vi "AddWatchdog.vi"(8 "error in (no error)":errorcluster, 10 "Watchdog":refnum<data-value>, 11 "Pound in":refnum<class "Pound.lvclass">) -> (0 "error out":errorcluster, 3 "Pound out":refnum<class "Pound.lvclass">)   [LabVIEW 2017, in "Pound.lvclass"]
doc: "Add a watchdog to the pack."
uses:
  <vilib>/NI/Software Watchdog/Pound/Pound.lvclass
  <vilib>/NI/Software Watchdog/Watchdog/Watchdog.lvclass
  <vilib>/NI/Software Watchdog/Pound/Pound.lvclass/Pound.ctl
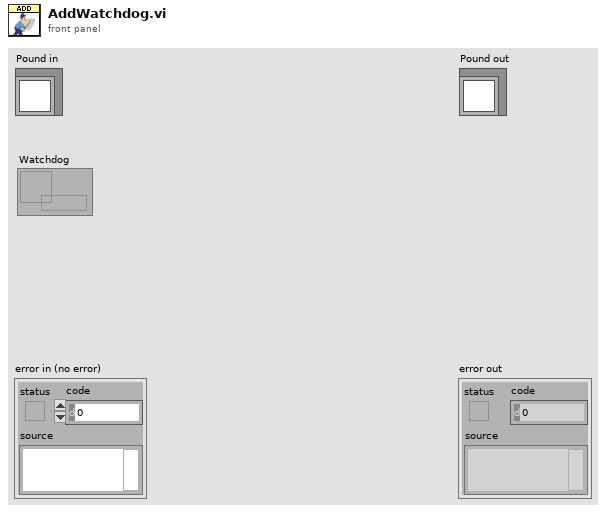
[diagram p1: front panel]
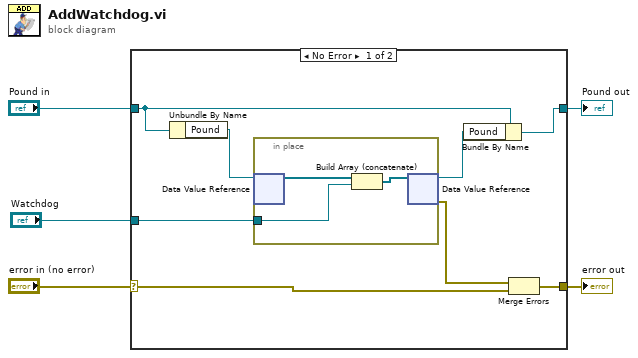
[diagram p0: block diagram]
diagram:
  n1 = case shown="No Error" "error in (no error)" {
    selector: "error in (no error)" -> [w6 w18]
    tunnel: [w8 w18] -> w4
    tunnel: [w10 w17] -> w2
    tunnel: "Pound in" -> [w11 w17]
    tunnel: "Watchdog" -> [w12 _]
    frame No Error {
      n2 = Unbundle By Name(w11) -> ("Pound"=w13:refnum<data-value>)
      n3 = in-place {
        in-place-border: w12 -> [w15]
        n4 = in-place-dvr #1(w13) -> (w14:refnum<data-value>[])  [unwired: 1 out]
        n5 = Build Array (concatenate)(w14, w15) -> (w16:refnum<data-value>[])
        n6 = in-place-dvr #1(w16) -> (w9:refnum<data-value>, w7:errorcluster)
      }
      n7 = Bundle By Name(cluster=w11, "Pound"=w9) -> (w10:refnum<class "Pound.lvclass">)
      n8 = Merge Errors(w7, w6) -> (w8:errorcluster)
    }
    frame Error {
    }
  }
  "error out" <- w4
  "Pound out" <- w2
